vi "Read CorrOffset File.vi"(8 "error in":errorcluster, 10 "CorrOffset File In":T1) -> (0 "error out":errorcluster, 2 "CorrOffset File Out":T1)   [LabVIEW 2020, in "GUCalibration2.lvlib"]
uses:
  GUCalibration2.lvlib
  <vilib>/regexp/Match Regular Expression.xnode
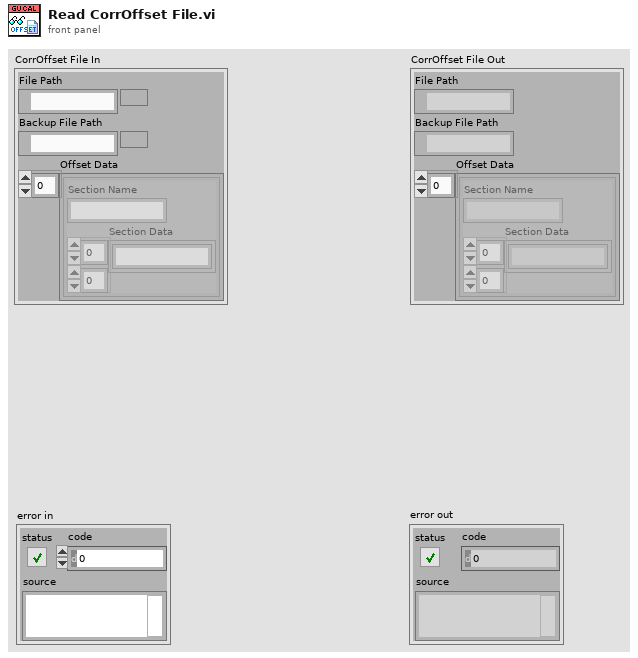
[diagram p1: front panel]
types:
  T1 = cluster{"File Path":path, "Backup File Path":path, "Offset Data":cluster{"Section Name":string, "Section Data":string[][]}[]}
  T2 = cluster{"Section Name":string, "Section Data":string[][]}[]
  T3 = cluster{"Section Name":string, "Section Data":string[][]}
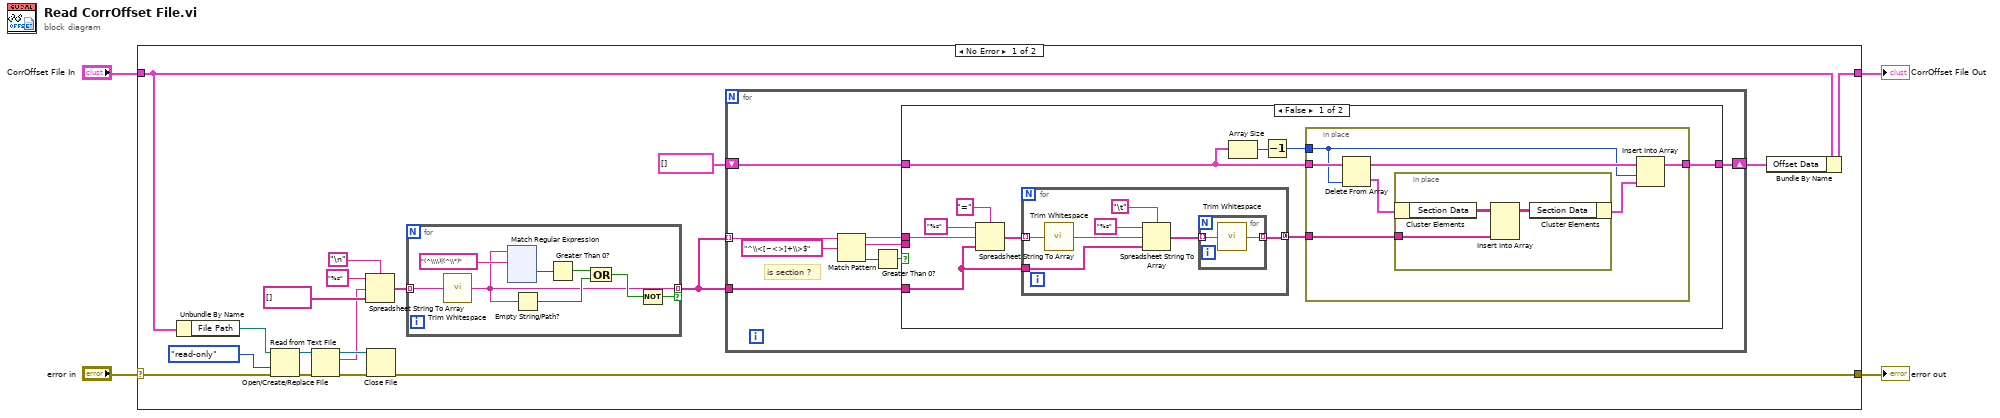
[diagram p0: block diagram]
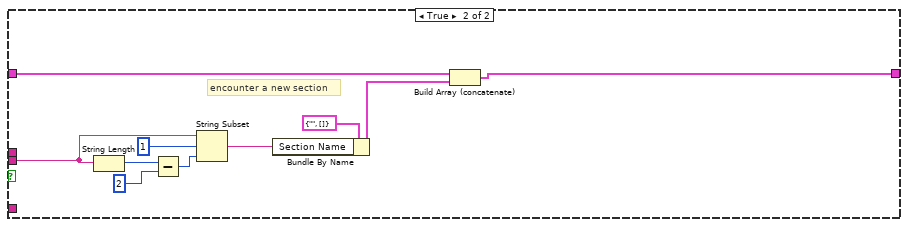
[diagram p2: hidden frame]
diagram:
  n1 = case shown="No Error" "error in" {
    selector: "error in" -> [w9 w193]
    tunnel: [w10 w193] -> w4
    tunnel: "CorrOffset File In" -> [w8 w194]
    tunnel: [w6 w194] -> w1
    frame No Error {
      n2 = Unbundle By Name(w8) -> ("File Path"=w5:path)
      n3 = Open/Create/Replace File(file path (use dialog)=w5, error in=w9, access (0:read/write)=enum16{"read/write", "read-only", "write-only"}."read-only") -> (refnum out=w20:refnum<file>, error out=w21:errorcluster)  [unwired: 3 in, 1 out]
      n4 = Read from Text File(file (use dialog)=w20, error in=w21) -> (refnum out=w18:refnum<file>, text=w14:string, error out=w19:errorcluster)  [unwired: 2 in, 1 out]
      n5 = Spreadsheet String To Array(delimiter (Tab)="\n", format string="%s", spreadsheet string=w14, array type (2D Dbl)=string[] []) -> (array=w22:string[])
      n6 = Close File(refnum=w18, error in=w19) -> (error out=w10:errorcluster)  [unwired: 1 out]
      n7 = for {
        tunnel: w22 -> [w78] mode=indexing
        tunnel: [w72] -> w11 mode=indexing if=w77
        n8 = call <vilib>:"Trim Whitespace.vi"("string"=w78) -> ("trimmed string"=w72:string)  [unwired: 1 in]
        n9 = xnode "Match Regular Expression"("input string"=w72, "regular expression"="(^\\\\)|(^\\*)") -> ("offset past match"=w71:i32)  [unwired: 4 in, 4 out]
        n10 = Empty String/Path?(string/path=w72) -> (empty?=w75:bool)
        n11 = Greater Than 0?(x=w71) -> (x > 0?=w74:bool)
        n12 = Compound Arithmetic op=OR(w74, w75) -> (w76:bool)
        n13 = Not(x=w76) -> (.not. x?=w77:bool)
      }
      n14 = for {
        tunnel: w11 -> [w30] mode=indexing
        tunnel: w11 -> [w31]
        shift-right: [w24] -> w7
        shift-left: T2 [] ("Config File") -> [w26]
        # "is section ?"
        n15 = Match Pattern(string=w30, regular expression="^\\<[~<>]+\\>$") -> (before substring=w23:string, match substring=w25:string, offset past match=w28:i32)  [unwired: 1 in, 1 out]
        n16 = Greater Than 0?(x=w28) -> (x > 0?=w27:bool)
        n17 = case shown="False" w27 {
          tunnel: w31 -> [w39 _]
          tunnel: w23 -> [w37 _]
          tunnel: w26 -> [w35 w63]
          tunnel: w25 -> [_ w68]
          tunnel: [w36 w61] -> w24
          frame False {
            n18 = Spreadsheet String To Array(delimiter (Tab)="=", format string="%s", spreadsheet string=w37, array type (2D Dbl)=w39) -> (array=w40:string[])
            n19 = for {
              tunnel: w40 -> [w56] mode=indexing
              tunnel: w39 -> [w58]
              tunnel: [w57] -> w32 mode=concatenating
              n20 = call <vilib>:"Trim Whitespace.vi"("string"=w56) -> ("trimmed string"=w55:string)  [unwired: 1 in]
              n21 = Spreadsheet String To Array(delimiter (Tab)="\t", format string="%s", spreadsheet string=w55, array type (2D Dbl)=w58) -> (array=w53:string[])
              n22 = for {
                tunnel: w53 -> [w60] mode=indexing
                tunnel: [w59] -> w57 mode=indexing
                n23 = call <vilib>:"Trim Whitespace.vi"("string"=w60) -> ("trimmed string"=w59:string)  [unwired: 1 in]
              }
            }
            n24 = Array Size(array=w35) -> (size(s)=w34:i32)
            n25 = Decrement(x=w34) -> (x-1=w33:i32)
            n26 = in-place {
              in-place-border: w35 -> [w48]
              in-place-border: w32 -> [w46]
              in-place-border: [w43] -> w36
              in-place-border: w33 -> [w42]
              n27 = Delete From Array(array=w48, index=w42) -> (deleted portion=w47:T3, array with subset deleted=w45:T2)  [unwired: 1 in]
              n28 = in-place {
                in-place-border: w46 -> [w51]
                n29 = in-place-cluster #1(w47) -> ("Section Data"=w50:string[][])
                n30 = Insert Into Array(array=w50, new element=w51) -> (w49:string[][])  [unwired: 2 in]
                n31 = in-place-cluster #1("Section Data"=w49) -> (w44:T3)
              }
              n32 = Insert Into Array(array=w45, index=w42, new element=w44) -> (w43:T2)
            }
          }
          frame True {
            # "encounter a new section"
            n33 = String Length(string=w68) -> (length=w67:i32)
            n34 = Subtract(x=w67, y=2) -> (x-y=w65:i32)
            n35 = String Subset(string=w68, offset (0)=1, length (rest)=w65) -> (substring=w64:string)
            n36 = Bundle By Name(cluster=T3 {"Section Name"="", "Section Data"=[]} ("Cluster"), "Section Name"=w64) -> (w62:T3)
            n37 = Build Array (concatenate)(w63, w62) -> (w61:T2)
          }
        }
      }
      n38 = Bundle By Name(cluster=w8, "Offset Data"=w7) -> (w6:T1)
    }
    frame Error {
    }
  }
  "error out" <- w4
  "CorrOffset File Out" <- w1
